vi "Step Type Not Supported--error.vi"(11 "Step Type":string) -> (0 "error out":errorcluster)   [LabVIEW 2020, in "MacroAssert.lvlib"]
uses:
  <vilib>/ErrorRing/Error Ring.xnode
  MacroAssert.lvlib
  <vilib>/Utility/error.llb/Error Cluster From Error Code.vi
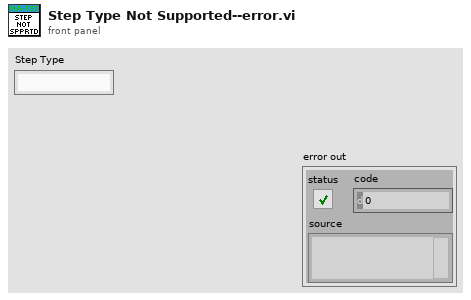
[diagram p1: front panel]
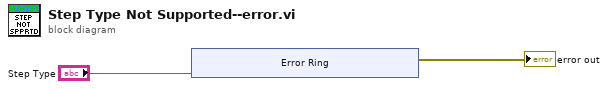
[diagram p0: block diagram]
diagram:
  n1 = xnode "Error Ring"("parameter 0"="Step Type") -> ("error out"=→"error out":errorcluster)
